vi "Get Caster Wheel Information.vi"(8 "error in (no error)":errorcluster, 11 "wheel in":refnum<class "NI_Robotics_Wheel.lvclass">) -> (0 "error out":errorcluster, 1 "wheel name":string, 2 "wheel parameters":T1={"wheel radius"=1.0, "gear ratio"=1.0, "forward rotation direction"=0} {"forward rotation direction" items=["Clockwise", "Counterclockwise"]}, 3 "wheel out":refnum<class "NI_Robotics_Wheel.lvclass">, 4 "motor communication":refnum<class "NI_Robotics_Motor Communication.lvclass">, 5 "caster parameters":T3={"forward offset"=0.0, "caster gear ratio"=1.0}, 6 "caster motor communication":refnum<class "NI_Robotics_Motor Communication.lvclass">)   [LabVIEW 2017, in "NI_Robotics_Wheel.lvclass"]
doc: "Returns information, such as <B>wheel radius</B> and <B>gear ratio</B>, for the wheel you specify. You must manually select the polymorphic instance to use."
uses:
  <vilib>/robotics/Steering/Wheel/NI_Robotics_Wheel.lvclass
  <vilib>/robotics/Steering/Caster Wheel/Caster Wheel Parameters.ctl
  <vilib>/robotics/Steering/Wheel/Wheel Parameters.ctl
  <vilib>/robotics/Steering/Wheel/Rotation Direction.ctl
  <vilib>/robotics/Actuation/Motor Communication/NI_Robotics_Motor Communication.lvclass
  <vilib>/robotics/Steering/Caster Wheel/NI_Robotics_Caster Wheel.lvclass
  c:/Program Files (x86)/National Instruments/LabVIEW 2017/vi.lib/robotics/Steering/Wheel/NI_Robotics_Wheel.lvclass
  <vilib>/robotics/Steering/Wheel/NI_Robotics_Wheel.lvclass/NI_Robotics_Wheel.ctl
  <vilib>/robotics/Steering/Caster Wheel/NI_Robotics_Caster Wheel.lvclass/NI_Robotics_Caster Wheel.ctl
  <vilib>/robotics/Steering/Wheel/Get Motor Communication.vi
  <vilib>/robotics/Steering/Wheel/Get Wheel Parameters.vi
  <vilib>/robotics/Steering/Caster Wheel/Get Caster Wheel Parameters.vi
  <vilib>/robotics/Utilities/Generate Error.vi
  <vilib>/robotics/Utilities/Clear Specific Error.vi
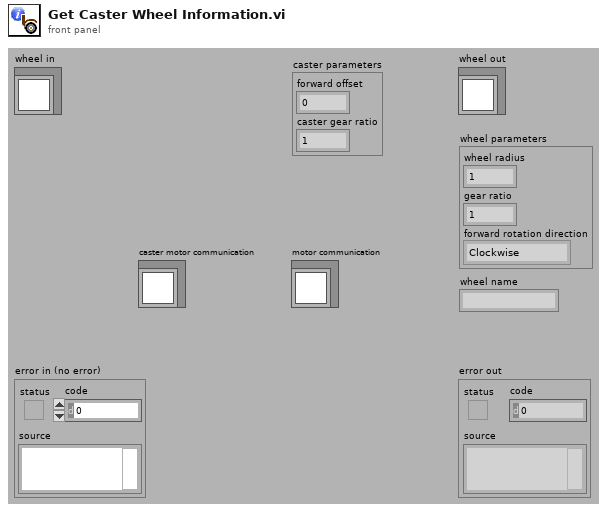
[diagram p1: front panel]
types:
  T1 = typedef "NI_Robotics_Wheel.lvclass/Wheel Parameters.ctl" = cluster{"wheel radius":dbl, "gear ratio":dbl, "forward rotation direction":T2}
  T2 = typedef "NI_Robotics_Wheel.lvclass/Rotation Direction.ctl" = u16
  T3 = typedef "NI_Robotics_Caster Wheel.lvclass/Caster Wheel Parameters.ctl" = cluster{"forward offset":dbl, "caster gear ratio":dbl}
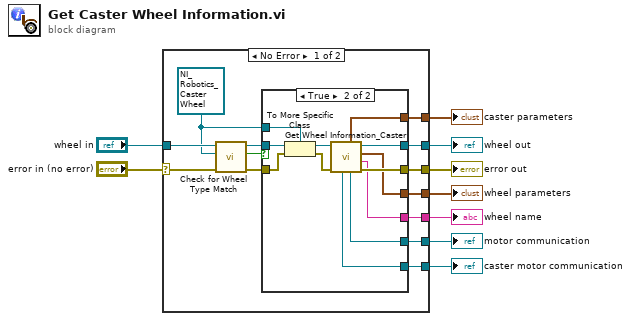
[diagram p0: block diagram]
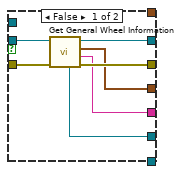
[diagram p2: hidden frame]
diagram:
  n1 = case shown="No Error" "error in (no error)" {
    selector: "error in (no error)" -> [w14 w43]
    tunnel: [w21 w43] -> w8
    tunnel: [w22 w42] -> w6
    tunnel: "wheel in" -> [w15 w42]
    tunnel: [w20 _] -> w5
    tunnel: [w19 _] -> w4
    tunnel: [w18 _] -> w3
    tunnel: [w17 _] -> w2
    tunnel: [w16 _] -> w1
    frame No Error {
      w10 = refnum<class "NI_Robotics_Caster Wheel.lvclass"> refnum ("caster wheel in")
      n2 = call <vilib>:"Check for Wheel Type Match.vi"("error in (no error)"=w14, "target wheel type"=w10, "wheel in"=w15) -> ("error out"=w11:errorcluster, "match?"=w12:bool, "wheel out"=w13:refnum<class "NI_Robotics_Wheel.lvclass">)  [unwired: 6 in]
      n3 = case shown="True" w12 {
        tunnel: w13 -> [w29 w34]
        tunnel: [w26 w41] -> w22
        tunnel: [w27 w40] -> w21
        tunnel: w10 -> [_ w32]
        tunnel: [_ w39] -> w20
        tunnel: [w25 w38] -> w19
        tunnel: [w24 w37] -> w18
        tunnel: [w23 w36] -> w17
        tunnel: [_ w35] -> w16
        tunnel: w11 -> [w28 w31]
        frame False {
          n4 = call <vilib>:"Get General Wheel Information.vi"("error in (no error)"=w28, "wheel in"=w29) -> ("error out"=w27:errorcluster, "wheel name"=w24:string, "wheel parameters"=w25:T1, "wheel out"=w26:refnum<class "NI_Robotics_Wheel.lvclass">, "motor communication"=w23:refnum<class "NI_Robotics_Motor Communication.lvclass">)  [unwired: 5 in]
        }
        frame True {
          n5 = To More Specific Class(target class=w32, reference=w34, error in=w31) -> (specific class reference=w33:refnum<class "NI_Robotics_Caster Wheel.lvclass">, error out=w30:errorcluster)
          n6 = call <vilib>:"Get Wheel Information_Caster.vi"("error in (no error)"=w30, "caster wheel in"=w33) -> ("error out"=w40:errorcluster, "wheel name"=w37:string, "wheel parameters"=w38:T1, "caster wheel out"=w41:refnum<class "NI_Robotics_Caster Wheel.lvclass">, "motor communication"=w36:refnum<class "NI_Robotics_Motor Communication.lvclass">, "caster parameters"=w39:T3, "caster motor communication"=w35:refnum<class "NI_Robotics_Motor Communication.lvclass">)  [unwired: 3 in]
        }
      }
    }
    frame Error {
    }
  }
  "error out" <- w8
  "wheel out" <- w6
  "caster parameters" <- w5
  "wheel parameters" <- w4
  "wheel name" <- w3
  "motor communication" <- w2
  "caster motor communication" <- w1
